vi "AssetInterface_Initalize Assets.vi"(8 "error in (no error)":errorcluster, 11 "Load in":refnum<class "Load.lvclass">) -> (0 "error out":errorcluster, 2 "TagDescriptions":refnum<class "tag descriptor.lvclass">[](array[class]), 3 "Load out":refnum<class "Load.lvclass">)   [LabVIEW 2015, in "Load.lvclass"]
uses:
  Load.lvclass
  <vilib>/NI/Tag Bus/tag/tag descriptor.lvclass
  TagBus/TagBus.lvclass
panel:
  out "Load_Status":cluster{"kW":dbl}
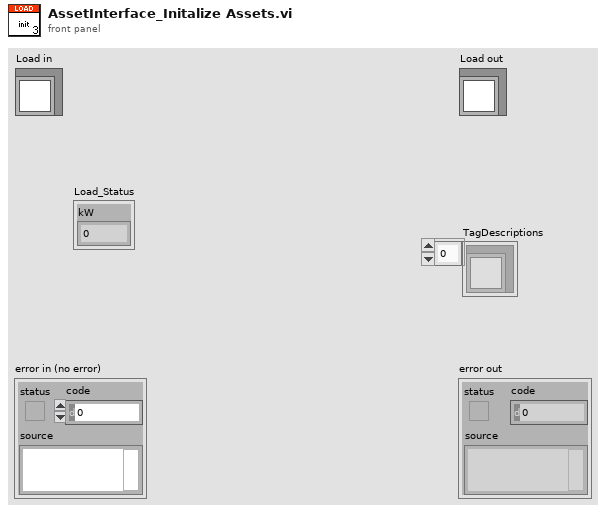
[diagram p1: front panel]
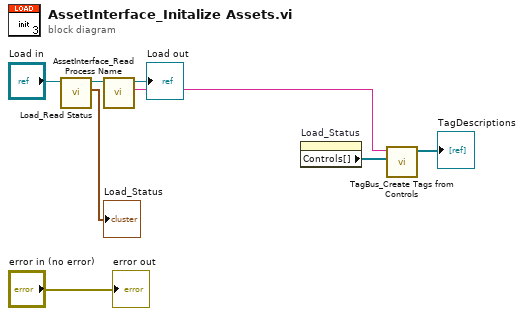
[diagram p0: block diagram]
diagram:
  n1 = call-dynamic "Load_Read Status.vi"("Load in"="Load in") -> ("Load_Status"=→"Load_Status":cluster{"kW":dbl}, "Load out"=w5:refnum<class "Load.lvclass">)  [unwired: 9 in]
  n2 = call-dynamic "AssetInterface_Read Process Name.vi"("Load in"=w5) -> ("Process Name"=w4:string, "Load out"=→"Load out":refnum<class "Load.lvclass">)  [unwired: 9 in]
  n3 = property on="Load_Status" class="Clust (strict)"() -> ("Controls[]"=w1:refnum<vi>[])  [unwired: 2 in, 2 out]
  n4 = call "TagBus_Create Tags from Controls.vi"("Array"=w1, "Process Name"=w4) -> ("TagDescriptions"=→"TagDescriptions":refnum<class "tag descriptor.lvclass">[])  [unwired: 9 in]
  "error out" <- "error in (no error)"
